vi "ttm_aecontrol_AEdata_read.vi"() -> ()   [LabVIEW 2010]
panel:
  out "Event(s)?":bool
  in  "Number of data points saved":i32=1000
  out "Sum of data points arrived within time window":dbl
  out "Time running (ms)":i32
  out "Array of last values":dbl[][](array[numeric])
  out "Last value received from data socket":dbl
  # "HUOM! MUISTA VAIHTAA timeWindow JAETUKSI MUUTTUJAKSI!"
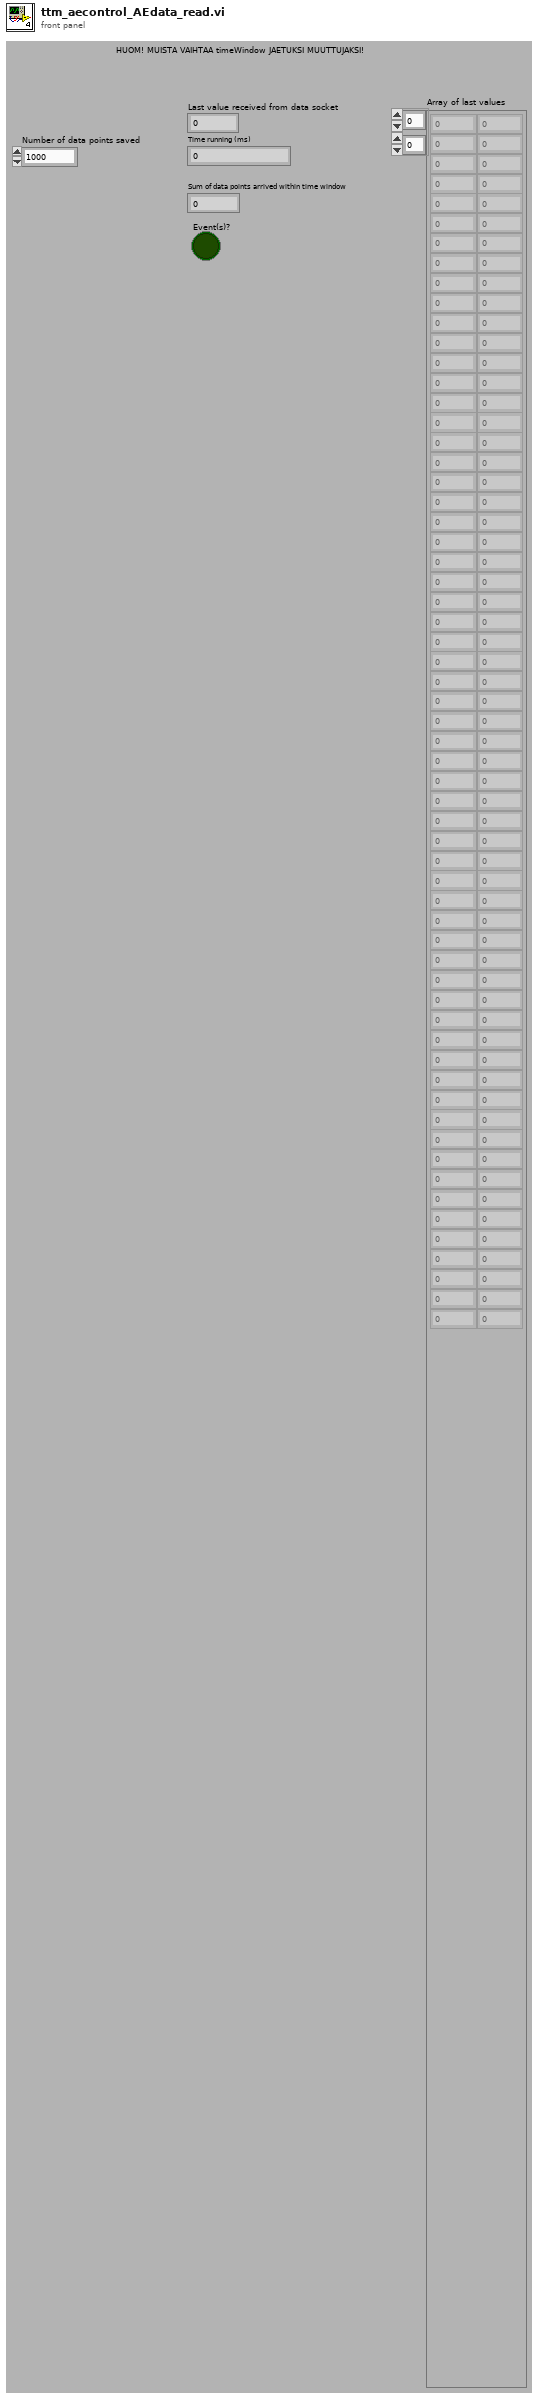
[diagram p1: front panel]
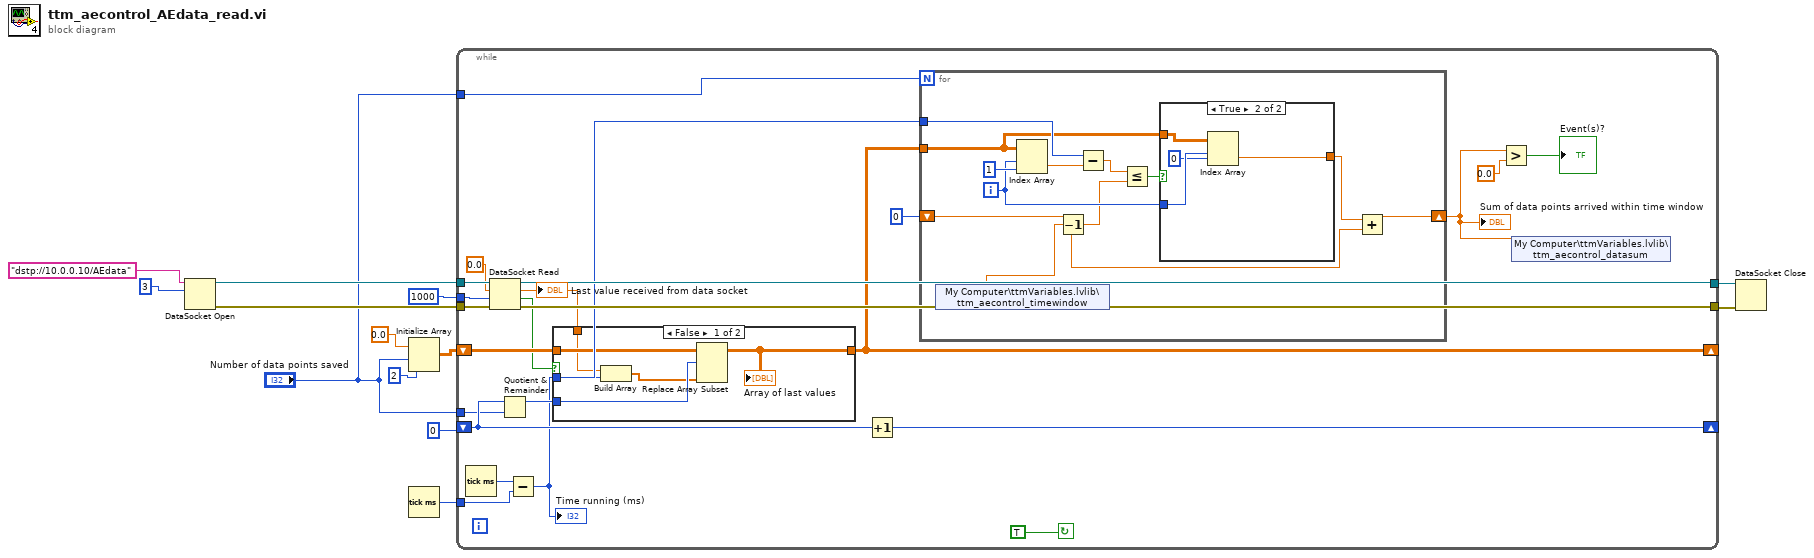
[diagram p0: block diagram]
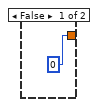
[diagram p3: hidden frame]
diagram:
  n1 = DataSocket Open(10:3, 11:"dstp://10.0.0.10/AEdata") -> (0:w10:errorcluster, 3:w11:refnum<k13>)  [unwired: 1 in, 1 out]
  n2 = Initialize Array(0.0, "Number of data points saved", 2) -> (w6:dbl[][])
  n3 = Tick Count (ms)() -> (millisecond timer value=w7:u32)
  n4 = while {
    tunnel: w11 -> [w36]
    tunnel: w10 -> [w35]
    tunnel: [w33] -> w9
    tunnel: [w32] -> w8
    tunnel: w7 -> [w29]
    shift-right: [w20] -> _
    shift-left: w6 -> [w28]
    shift-right: [w27] -> _
    shift-left: 0 -> [w26]
    tunnel: "Number of data points saved" -> [w25]
    tunnel: "Number of data points saved" -> [w22]
    tunnel: 1000 -> [w17]
    stop <- TRUE continue-if-true
    n5 = Tick Count (ms)() -> (millisecond timer value=w31:u32)
    n6 = DataSocket Read(8:w35, 9:w17, 10:0.0, 11:w36) -> (0:w32:errorcluster, 1:w18:bool, 2:w23:dbl, 3:w33:refnum<k13>)  [unwired: 4 out]
    "Last value received from data socket" <- w23
    n7 = Quotient & Remainder(x=w26, y=w25) -> (x-y*floor(x/y)=w24:i32)  [unwired: 1 out]
    n8 = Subtract(x=w31, y=w29) -> (x-y=w21:u32)
    "Time running (ms)" <- w21
    n9 = case shown="False" w18 {
      tunnel: w28 -> [w42 w43]
      tunnel: w24 -> [w41 _]
      tunnel: w23 -> [w40 _]
      tunnel: w21 -> [w39 _]
      tunnel: [w37 w43] -> w20
      frame False {
        n10 = Build Array(w40, w39) -> (w38:dbl[])
        n11 = Replace Array Subset(array=w42, new element=w38, index (row)=w41) -> (w37:dbl[][])  [unwired: 1 in]
        "Array of last values" <- w37
      }
      frame True {
      }
    }
    n12 = Increment(x=w26) -> (x+1=w27:i32)
    n13 = for {
      N: w22 -> [_]
      tunnel: w21 -> [w54]
      tunnel: w20 -> [w50]
      shift-right: [w46] -> w16
      shift-left: 0 -> [w47]
      i -> [w49]
      n14 = shared-variable "My Computer\\ttmVariables.lvlib\\ttm_aecontrol_timewindow"() -> (w44:dbl)  [unwired: 1 in, 1 out]
      n15 = Index Array(array=w50, index (row)=w49, index (col)=1) -> (element=w53:dbl)
      n16 = Decrement(x=w44) -> (x-1=w45:dbl)
      n17 = Subtract(x=w54, y=w53) -> (x-y=w51:dbl)
      n18 = Less Or Equal?(x=w51, y=w45) -> (x <= y?=w52:bool)
      n19 = case shown="True" w52 {
        tunnel: w50 -> [_ w60]
        tunnel: w49 -> [_ w59]
        tunnel: [0 w57] -> w48
        frame False {
        }
        frame True {
          n20 = Index Array(array=w60, index (row)=w59, index (col)=0) -> (element=w57:dbl)
        }
      }
      n21 = Add(x=w48, y=w47) -> (x+y=w46:dbl)
    }
    "Sum of data points arrived within time window" <- w16
    n22 = Greater?(x=w16, y=0.0) -> (0:→"Event(s)?":bool)
    n23 = shared-variable "My Computer\\ttmVariables.lvlib\\ttm_aecontrol_datasum"(w16) -> ()  [unwired: 1 in, 1 out]
  }
  n24 = DataSocket Close(8:w8, 11:w9) -> ()  [unwired: 3 out]
